vi "rtndata.vi"(0 "object in":refnum<class "212format_work.lvclass">, 1 "in":T1, 5 "error in (no error)":errorcluster) -> (14 "object out":refnum<class "212format_work.lvclass">, 15 "out":T2, 19 "error out":errorcluster)   [LabVIEW 2016, in "212format_work.lvclass"]
uses:
  212format_work.lvclass
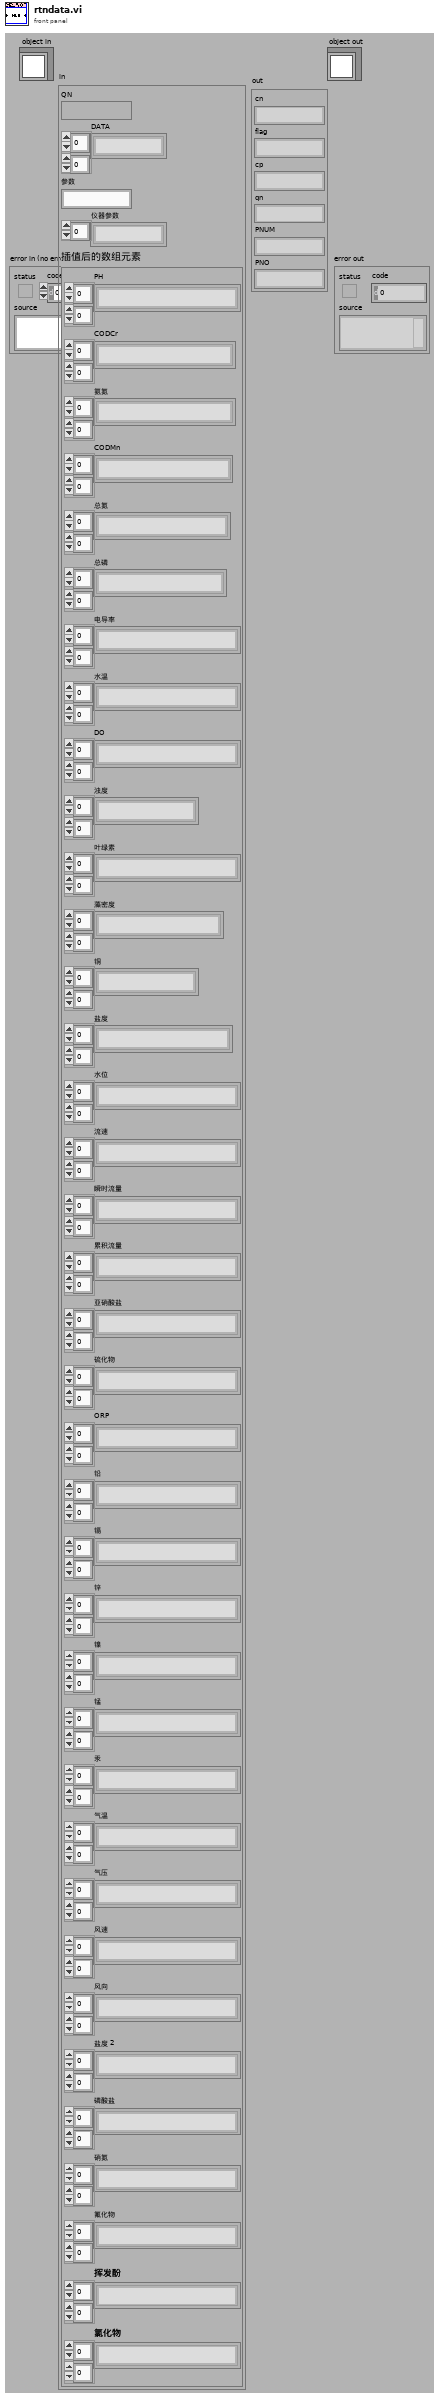
[diagram p1: front panel]
types:
  T1 = cluster{"QN":string, "DATA":string[][], "参数":string, "仪器参数":string[], "插值后的数组元素":cluster{"PH":string[][], "CODCr":string[][], "氨氮":string[][], "CODMn":string[][], "总氮":string[][], "总磷":string[][], "电导率":string[][], "水温":string[][], "DO":string[][], "浊度":string[][], "叶绿素":string[][], "藻密度":string[][], "铜":string[][], "盐度":string[][], "水位":string[][], "流速":string[][], "瞬时流量":string[][], "累积流量":string[][], "亚硝酸盐":string[][], "硫化物":string[][], "ORP":string[][], "铅":string[][], "镉":string[][], "锌":string[][], "镍":string[][], "锰":string[][], "汞":string[][], "气温":string[][], "气压":string[][], "风速":string[][], "风向":string[][], "盐度 2":string[][], "磷酸盐":string[][], "硝氮":string[][], "氟化物":string[][], "挥发酚":string[][], "氯化物":string[][]}}
  T2 = cluster{"cn":string, "flag":string, "cp":string, "qn":string, "PNUM":string, "PNO":string}
  T3 = enum16{"小时数据", "实时数据", "平行样测试", "集成干预测试", "加标回收测试", "核查数据", "空白零点跨度数据", "提取小时数据", "提取实时数据", "操作日志", "仪器参数", "3090仪器参数", "提取仪器参数", "报警信息"}
  T4 = enum16{"formattime", "formatminute", "formathour"}
  T5 = typedef "212format_work.lvclass/interdata控件.ctl" = cluster{"数据发送协议":enum16{"2005-212协议", "2017-212协议"}, "枚举":enum16{"返回请求应答", "上传数据", "返回执行结果"}, "系统编码ST":string, "主动上报数据中":bool, "数据组合发送":bool, "地表水/污染源":bool, "应用环境":enum16{"STD", "GB212"}}
  T6 = typedef "212format_work.lvclass/data控件.ctl" = cluster{"选择发送的参数":string, "插值后的数组元素":cluster{"PH":string[][], "CODCr":string[][], "氨氮":string[][], "CODMn":string[][], "总氮":string[][], "总磷":string[][], "电导率":string[][], "水温":string[][], "DO":string[][], "浊度":string[][], "叶绿素":string[][], "藻密度":string[][], "铜":string[][], "盐度":string[][], "水位":string[][], "流速":string[][], "瞬时流量":string[][], "累积流量":string[][], "亚硝酸盐":string[][], "硫化物":string[][], "ORP":string[][], "铅":string[][], "镉":string[][], "锌":string[][], "镍":string[][], "锰":string[][], "汞":string[][], "气温":string[][], "气压":string[][], "风速":string[][], "风向":string[][], "盐度 2":string[][], "磷酸盐":string[][], "硝氮":string[][], "氟化物":string[][], "挥发酚":string[][], "氯化物":string[][]}, "register values":u16[], "columns输出":string[], "环境参数":string[][], "仪器编码":string, "实时数据发送间隔":u32, "实时数据参数":string, "参数系数簇":cluster{"CODMn":dbl, "CODCr":dbl, "DO":dbl, "铜":dbl, "PH":dbl, "氨氮":dbl, "比电导率":dbl, "水温":dbl, "COD":dbl, "浊度":dbl, "总氮":dbl, "总磷":dbl, "叶绿素a":dbl, "藻密度":dbl, "水位":dbl, "流速":dbl, "瞬时流量":dbl, "累积流量":dbl, "亚硝酸盐":dbl, "硫化物":dbl, "ORP":dbl, "铅":dbl, "镉":dbl, "锌":dbl, "镍":dbl, "锰":dbl, "汞":dbl, "气温":dbl, "气压":dbl, "风速":dbl, "风向":dbl, "盐度":dbl, "磷酸盐":dbl, "硝氮":dbl, "氟化物":dbl, "挥发酚":dbl, "氯化物":dbl}, "因子编码簇":cluster{"CODMn":string, "CODCr":string, "DO":string, "铜":string, "PH":string, "氨氮":string, "比电导率":string, "水温":string, "COD":string, "浊度":string, "总氮":string, "总磷":string, "叶绿素a":string, "藻密度":string, "水位":string, "流速":string, "瞬时流量":string, "累积流量":string, "亚硝酸盐":string, "硫化物":string, "ORP":string, "铅":string, "镉":string, "锌":string, "镍":string, "锰":string, "汞":string, "气温":string, "气压":string, "风速":string, "风向":string, "盐度":string, "磷酸盐":string, "硝氮":string, "氟化物":string, "挥发酚":string, "氯化物":string}, "小时数据发送次数":i32, "读取试剂余量的值":u16[], "参数编码":string, "数据数组大小":i32, "总包数":i32, "当前包号":i32, "columns":string[], "剖面多参数":string[][], "分包标准":i32}
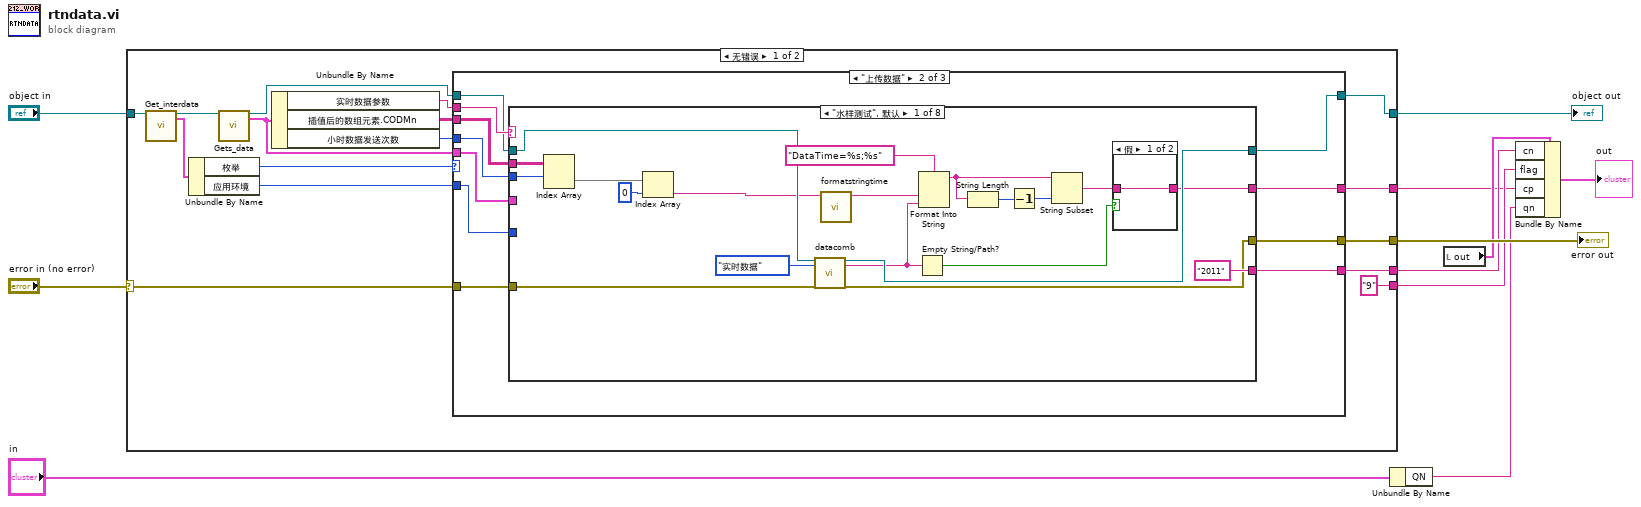
[diagram p0: block diagram]
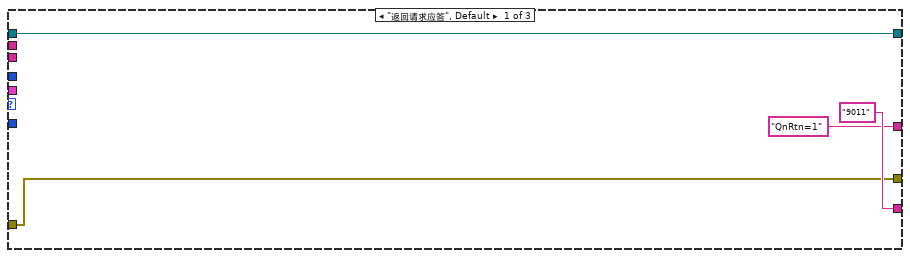
[diagram p2: hidden frame]
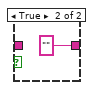
[diagram p3: hidden frame]
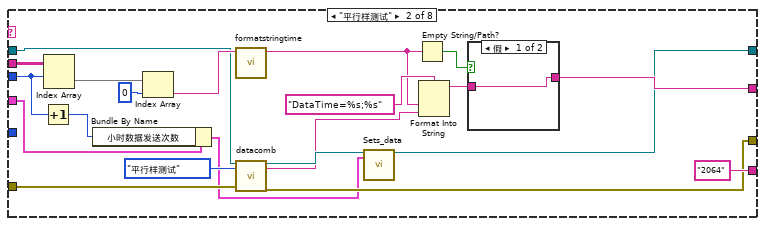
[diagram p4: hidden frame]
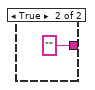
[diagram p5: hidden frame]
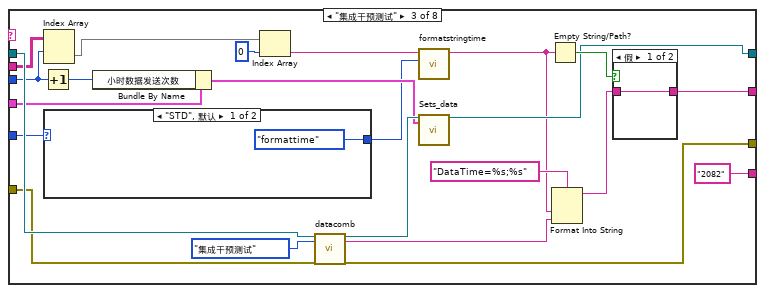
[diagram p6: hidden frame]
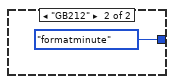
[diagram p7: hidden frame]
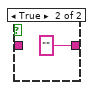
[diagram p8: hidden frame]
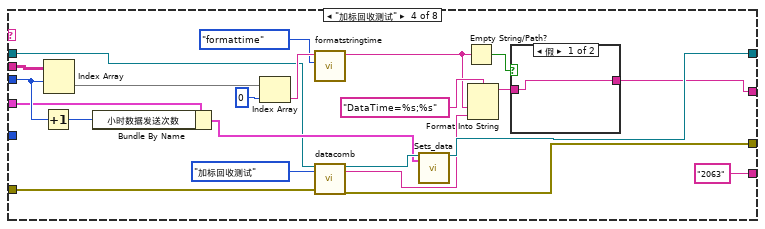
[diagram p9: hidden frame]
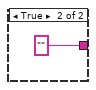
[diagram p10: hidden frame]
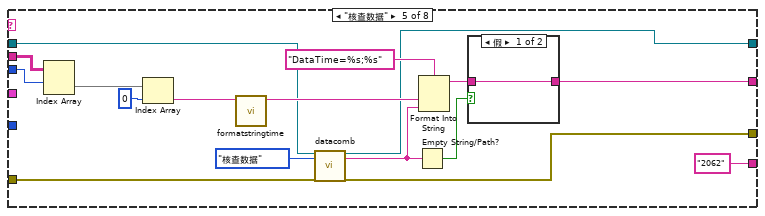
[diagram p11: hidden frame]
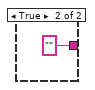
[diagram p12: hidden frame]
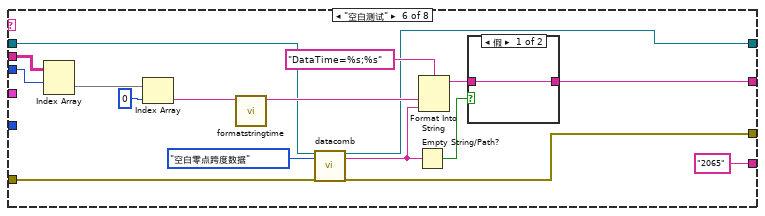
[diagram p13: hidden frame]
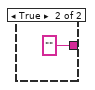
[diagram p14: hidden frame]
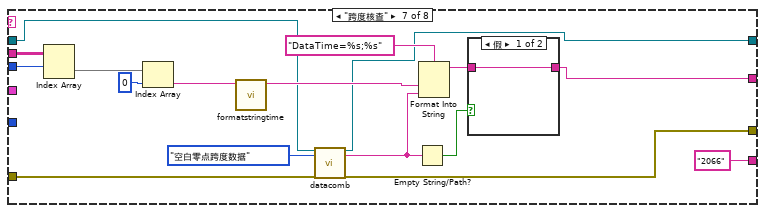
[diagram p15: hidden frame]
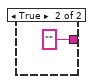
[diagram p16: hidden frame]
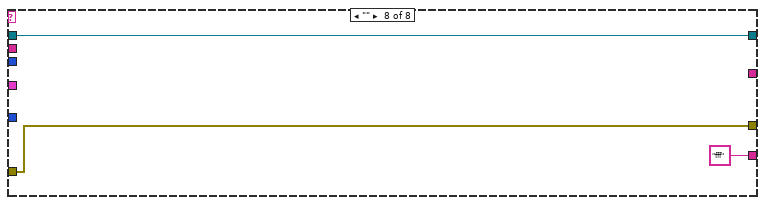
[diagram p17: hidden frame]
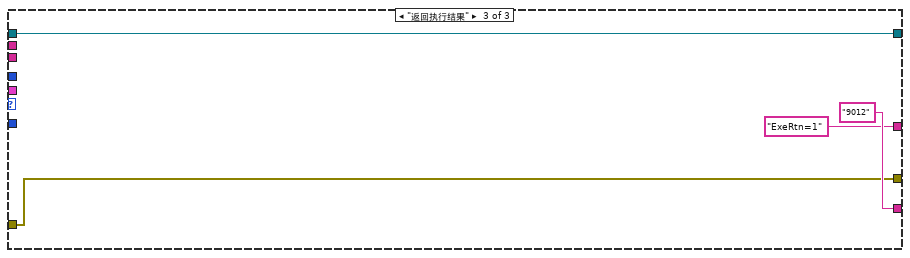
[diagram p18: hidden frame]
diagram:
  n1 = case shown="无错误" "error in (no error)" {
    selector: "error in (no error)" -> [w17 w204]
    tunnel: [w16 w204] -> w10
    tunnel: [w18 w203] -> w8
    tunnel: "object in" -> [w26 w203]
    tunnel: [w21 _] -> w3
    tunnel: [w23 _] -> w5
    tunnel: ["9" ("ST") _] -> w4
    frame No Error {
      n2 = call-dynamic "Get_interdata.vi"("object in"=w26) -> ("object out"=w22:refnum<class "212format_work.lvclass">, "interdata"=w25:T5)  [unwired: 16 in, 1 out]
      n3 = Unbundle By Name(w25) -> ("枚举"=w24:enum16{"返回请求应答", "上传数据", "返回执行结果"}, "应用环境"=w12:enum16{"STD", "GB212"})
      n4 = call-dynamic "Gets_data.vi"("object in"=w22) -> ("object out"=w19:refnum<class "212format_work.lvclass">, "data"=w13:T6)  [unwired: 16 in, 1 out]
      n5 = Unbundle By Name(w13) -> ("实时数据参数"=w20:string, "插值后的数组元素.CODMn"=w15:string[][], "小时数据发送次数"=w14:i32)
      n6 = case shown="\"上传数据\"" w24 {
        tunnel: ["9011" ("CN") w41 "9012" ("CN")] -> w23
        tunnel: ["QnRtn=1" w38 "ExeRtn=1"] -> w21
        tunnel: w20 -> [_ w42 _]
        tunnel: w19 -> [w29 w40 w199]
        tunnel: [w29 w39 w199] -> w18
        tunnel: w17 -> [w28 w37 w200]
        tunnel: [w28 w36 w200] -> w16
        tunnel: w15 -> [_ w35 _]
        tunnel: w14 -> [_ w34 _]
        tunnel: w13 -> [_ w33 _]
        tunnel: w12 -> [_ w32 _]
        frame "返回请求应答", Default {
        }
        frame "上传数据" {
          n7 = case shown="\"水样测试\", 默认" w42 {
            tunnel: ["2011" ("CN") "2064" ("CN") "2082" ("CN") "2063" ("CN") "2062" ("CN") "2065" ("CN") "2066" ("CN") "fff" ("CN")] -> w41
            tunnel: w40 -> [w60 w75 w97 w121 w145 w163 w182 w197]
            tunnel: [w59 w68 w99 w120 w143 w164 w183 w197] -> w39
            tunnel: [w45 w78 w100 w119 w141 w160 w178 _] -> w38
            tunnel: w37 -> [w58 w76 w96 w122 w144 w162 w181 w196]
            tunnel: [w57 w77 w98 w118 w142 w161 w177 w196] -> w36
            tunnel: w35 -> [w54 w74 w94 w124 w147 w159 w180 _]
            tunnel: w34 -> [w53 w73 w93 w125 w146 w158 w179 _]
            tunnel: w33 -> [_ w72 w95 w123 _ _ _ _]
            tunnel: w32 -> [_ _ w91 _ _ _ _ _]
            frame "水样测试", Default {
              n8 = Index Array(array=w54, index (row)=w53) -> (element=w56:string[])  [unwired: 1 in]
              n9 = Index Array(array=w56, index=0 ("索引")) -> (element=w52:string)
              n10 = call-dynamic "datacomb.vi"("object in"=w60, "枚举"=T3."实时数据", "error in (no error)"=w58) -> ("object out"=w59:refnum<class "212format_work.lvclass">, "字符串"=w44:string, "error out"=w57:errorcluster)  [unwired: 14 in]
              n11 = call "formatstringtime.vi"("字符串"=w52) -> ("result string"=w46:string)  [unwired: 10 in]
              n12 = Empty String/Path?(string/path=w44) -> (empty?=w47:bool)
              n13 = Format Into String(format string="DataTime=%s;%s", w46, w44) -> (resulting string=w43:string)  [unwired: 2 in, 1 out]
              n14 = String Length(string=w43) -> (length=w49:i32)
              n15 = Decrement(x=w49) -> (x-1=w50:i32)
              n16 = String Subset(string=w43, length (rest)=w50) -> (substring=w51:string)  [unwired: 1 in]
              n17 = case shown="假" w47 {
                tunnel: [w63 ""] -> w45
                tunnel: w51 -> [w63 _]
                frame False {
                }
                frame True {
                }
              }
            }
            frame "平行样测试" {
              n18 = Increment(x=w73) -> (x+1=w71:i32)
              n19 = Index Array(array=w74, index (row)=w73) -> (element=w83:string[])  [unwired: 1 in]
              n20 = Bundle By Name(cluster=w72, "小时数据发送次数"=w71) -> (w70:T6)
              n21 = Index Array(array=w83, index=0 ("索引")) -> (element=w81:string)
              n22 = call "formatstringtime.vi"("字符串"=w81) -> ("result string"=w65:string)  [unwired: 10 in]
              n23 = call-dynamic "datacomb.vi"("object in"=w75, "枚举"=T3."平行样测试", "error in (no error)"=w76) -> ("object out"=w69:refnum<class "212format_work.lvclass">, "字符串"=w67:string, "error out"=w77:errorcluster)  [unwired: 14 in]
              n24 = call-dynamic "Sets_data.vi"("object in"=w69, "data"=w70) -> ("object out"=w68:refnum<class "212format_work.lvclass">)  [unwired: 16 in, 1 out]
              n25 = Empty String/Path?(string/path=w65) -> (empty?=w79:bool)
              n26 = Format Into String(format string="DataTime=%s;%s", w65, w67) -> (resulting string=w66:string)  [unwired: 2 in, 1 out]
              n27 = case shown="假" w79 {
                tunnel: [w86 ""] -> w78
                tunnel: w66 -> [w86 _]
                frame False {
                }
                frame True {
                }
              }
            }
            frame "集成干预测试" {
              n28 = Increment(x=w93) -> (x+1=w107:i32)
              n29 = Index Array(array=w94, index (row)=w93) -> (element=w102:string[])  [unwired: 1 in]
              n30 = case shown="\"STD\", 默认" w91 {
                tunnel: [T4."formattime" ("枚举") T4."formatminute" ("枚举")] -> w92
                frame "STD", Default {
                }
                frame "GB212" {
                }
              }
              n31 = Bundle By Name(cluster=w95, "小时数据发送次数"=w107) -> (w108:T6)
              n32 = Index Array(array=w102, index=0 ("索引")) -> (element=w104:string)
              n33 = call-dynamic "datacomb.vi"("object in"=w97, "枚举"=T3."集成干预测试", "error in (no error)"=w96) -> ("object out"=w109:refnum<class "212format_work.lvclass">, "字符串"=w90:string, "error out"=w98:errorcluster)  [unwired: 14 in]
              n34 = call "formatstringtime.vi"("枚举"=w92, "字符串"=w104) -> ("result string"=w88:string)  [unwired: 9 in]
              n35 = call-dynamic "Sets_data.vi"("object in"=w109, "data"=w108) -> ("object out"=w99:refnum<class "212format_work.lvclass">)  [unwired: 16 in, 1 out]
              n36 = Empty String/Path?(string/path=w88) -> (empty?=w106:bool)
              n37 = Format Into String(format string="DataTime=%s;%s", w88, w90) -> (resulting string=w89:string)  [unwired: 2 in, 1 out]
              n38 = case shown="假" w106 {
                tunnel: [w113 ""] -> w100
                tunnel: w89 -> [w113 _]
                frame False {
                }
                frame True {
                }
              }
            }
            frame "加标回收测试" {
              n39 = Increment(x=w125) -> (x+1=w133:i32)
              n40 = Index Array(array=w124, index (row)=w125) -> (element=w128:string[])  [unwired: 1 in]
              n41 = Bundle By Name(cluster=w123, "小时数据发送次数"=w133) -> (w134:T6)
              n42 = Index Array(array=w128, index=0 ("索引")) -> (element=w130:string)
              n43 = call "formatstringtime.vi"("枚举"=T4."formattime", "字符串"=w130) -> ("result string"=w115:string)  [unwired: 9 in]
              n44 = call-dynamic "datacomb.vi"("object in"=w121, "枚举"=T3."加标回收测试", "error in (no error)"=w122) -> ("object out"=w135:refnum<class "212format_work.lvclass">, "字符串"=w117:string, "error out"=w118:errorcluster)  [unwired: 14 in]
              n45 = call-dynamic "Sets_data.vi"("object in"=w135, "data"=w134) -> ("object out"=w120:refnum<class "212format_work.lvclass">)  [unwired: 16 in, 1 out]
              n46 = Empty String/Path?(string/path=w115) -> (empty?=w132:bool)
              n47 = Format Into String(format string="DataTime=%s;%s", w115, w117) -> (resulting string=w116:string)  [unwired: 2 in, 1 out]
              n48 = case shown="假" w132 {
                tunnel: [w137 ""] -> w119
                tunnel: w116 -> [w137 _]
                frame False {
                }
                frame True {
                }
              }
            }
            frame "核查数据" {
              n49 = Index Array(array=w147, index (row)=w146) -> (element=w153:string[])  [unwired: 1 in]
              n50 = Index Array(array=w153, index=0 ("索引")) -> (element=w151:string)
              n51 = call "formatstringtime.vi"("字符串"=w151) -> ("result string"=w148:string)  [unwired: 10 in]
              n52 = call-dynamic "datacomb.vi"("object in"=w145, "枚举"=T3."核查数据", "error in (no error)"=w144) -> ("object out"=w143:refnum<class "212format_work.lvclass">, "字符串"=w140:string, "error out"=w142:errorcluster)  [unwired: 14 in]
              n53 = Empty String/Path?(string/path=w140) -> (empty?=w149:bool)
              n54 = Format Into String(format string="DataTime=%s;%s", w148, w140) -> (resulting string=w139:string)  [unwired: 2 in, 1 out]
              n55 = case shown="假" w149 {
                tunnel: [w156 ""] -> w141
                tunnel: w139 -> [w156 _]
                frame False {
                }
                frame True {
                }
              }
            }
            frame "空白测试" {
              n56 = Index Array(array=w159, index (row)=w158) -> (element=w172:string[])  [unwired: 1 in]
              n57 = Index Array(array=w172, index=0 ("索引")) -> (element=w170:string)
              n58 = call "formatstringtime.vi"("字符串"=w170) -> ("result string"=w167:string)  [unwired: 10 in]
              n59 = call-dynamic "datacomb.vi"("object in"=w163, "枚举"=T3."空白零点跨度数据", "error in (no error)"=w162) -> ("object out"=w164:refnum<class "212format_work.lvclass">, "字符串"=w166:string, "error out"=w161:errorcluster)  [unwired: 14 in]
              n60 = Empty String/Path?(string/path=w166) -> (empty?=w168:bool)
              n61 = Format Into String(format string="DataTime=%s;%s", w167, w166) -> (resulting string=w165:string)  [unwired: 2 in, 1 out]
              n62 = case shown="假" w168 {
                tunnel: [w175 ""] -> w160
                tunnel: w165 -> [w175 _]
                frame False {
                }
                frame True {
                }
              }
            }
            frame "跨度核查" {
              n63 = Index Array(array=w180, index (row)=w179) -> (element=w191:string[])  [unwired: 1 in]
              n64 = Index Array(array=w191, index=0 ("索引")) -> (element=w189:string)
              n65 = call "formatstringtime.vi"("字符串"=w189) -> ("result string"=w186:string)  [unwired: 10 in]
              n66 = call-dynamic "datacomb.vi"("object in"=w182, "枚举"=T3."空白零点跨度数据", "error in (no error)"=w181) -> ("object out"=w183:refnum<class "212format_work.lvclass">, "字符串"=w185:string, "error out"=w177:errorcluster)  [unwired: 14 in]
              n67 = Empty String/Path?(string/path=w185) -> (empty?=w187:bool)
              n68 = Format Into String(format string="DataTime=%s;%s", w186, w185) -> (resulting string=w184:string)  [unwired: 2 in, 1 out]
              n69 = case shown="假" w187 {
                tunnel: [w194 ""] -> w178
                tunnel: w184 -> [w194 _]
                frame False {
                }
                frame True {
                }
              }
            }
            frame "" {
            }
          }
        }
        frame "返回执行结果" {
        }
      }
    }
    frame Error {
    }
  }
  "error out" <- w10
  "object out" <- w8
  n70 = Unbundle By Name("in") -> ("QN"=w1:string)
  n71 = local read "out"() -> (w7:T2)
  n72 = Bundle By Name(cluster=w7, "cn"=w5, "flag"=w4, "cp"=w3, "qn"=w1) -> (→"out":T2)
